vi "GenericDriveIO.vi"(0 "GenericDriveCommand":T1="DePowerMotor", 2 "Channel Name":string, 4 "String Value":string, 6 "Numeric Value":dbl format="%.2f", 8 "Address":u8, 9 "Type":string="ParkerX", 10 "Port Name":string) -> (5 "String Reply":string, 7 "Numeric Reply":sgl format="%.2f")   [LabVIEW 2014]
uses:
  GenericDriveCommand.ctl
  PARKER X/X-_commands.ctl
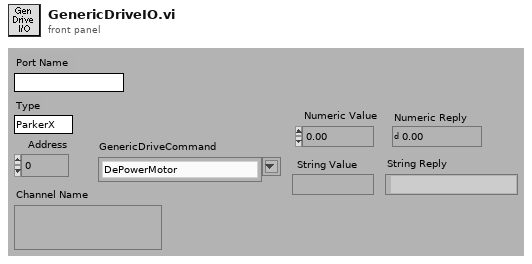
[diagram p1: front panel]
types:
  T1 = typedef "GenericDriveCommand.ctl" = string
  T2 = typedef "X-_commands.ctl" = enum16{"A-    Acceleration (rps)", "B-    Buffer Status", "C-    Continue", "CG-  Correction Gain", "CR-  Cariage Return", "D-    Distance (pulses)", "DB-  Dead Band (encoder steps)", "DW- Deadband Window (encoder steps)", "E-    Enable Communications", "ER-  Encoder Resolution (steps/rev)", "F-    Disable Communications", "FS-  Encoder Functions Report", "FSA- Incremental/Absolute (0/1)", "FSB- Motor/Encoder Step Mode (0/1)", "FSC- Enable/Disable Position Maint. (1/0)", "FSD- Stop/Continue on Stall (1/0)", "FSE- Activate o/p1 on Stall (1/0)", "FSF- Stop Motion on Trig3 (1/0)", "FSG- Activate o/p2 in Deadband (1/0)", "FSH- Enable Stall Detect (1/0)", "G- Go", "GH- Go Home and Zero (+/-V)", "^H- Delete ", "H- Direction Reverse/CCW/CW (0,1,2)", "IS- Input Status", "K- Kill", "L- Loop (n)", "LD- Limit DISABLE (0-none,1-CW,2-CCW,3-Both)", "LF- Line Feed", "MC- Mode Continuous", "MN- Mode Normal", "MPA- Motor Postion Absolute", "MPI- Motor Position Incremental", "MR- Motor Resolution (Drive Steps/rev)", "N- End of Loop", "O- Output (00,01,10,11)", "OS- Report Homing Setup", "OSA- NO/NC Limits (1/0)", "OSB- Back Up to Home/Edge? (0/1)", "OSC- NO/NC Home Switch (1/0)", "OSD- Enable Encoder Z for Home (0/1)", "OSH- Reference Edge for Home CW/CCW (0/1)", "PR- Report ABSOLUTE Position", "PS- Pause until Continue", "PX- Report Absolute ENCODER Position", "PZ- Zero Absolute Counter", "\"- Quote (17 ASCII +Space)", "Q- Enter/Exit Velocity Profiling (1/0)", "R- Request Indexer Status", "RA- Report Limit Switch Status", "RB- Report Loop, Pause, Shutdown, Trigger Status", "RC- Report Closed Loop Status", "RM- Velocity Streaming Rate Multiplier (000-FFF)", "RV- Report Revision Level", "S- Controlled Stop", "SN- Debounce (1-1000ms)", "SS- Report Software Switch Status", "SSA- Disable RS232 Echo (1/0)", "SSG- Clear/Save Command Buffer on Limit (0/1)", "SSH- Clear/Save Command Buffer on Stop (0/1)", "ST- Shutdown (1/0)", "SV- Servoing Setting (0,1,2,3)", "T- Time Delay (0.01-99999.99)", "TR- Wait for Trigger High/Low/Ignore (1/0/X)", "TS- Report Trigger Status", "U- Pause after Move Until Continue", "V- Velocity (0.01-50.00 revs/sec)", "W1- Report Relative Position <Signed Binary>", "W3- Report Relative Position <Hexadecimal>", "Y- Abort Loop at N", "Z-    Reset to Defaults", "#-    Disable/Set Soft Addresses (0/1-255)"}
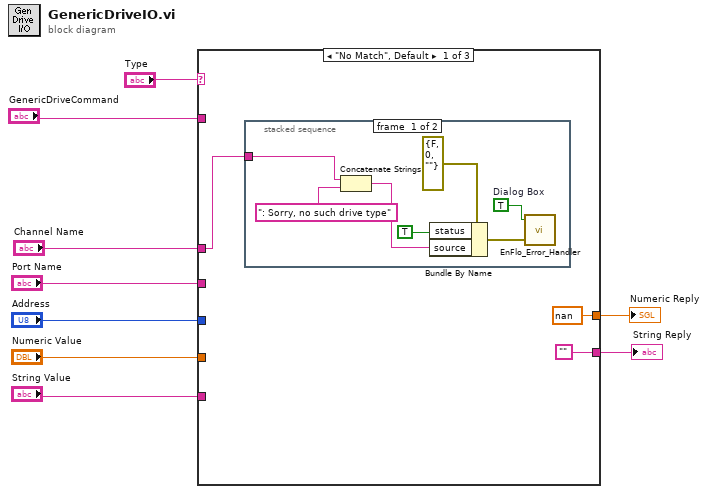
[diagram p0: block diagram]
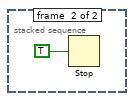
[diagram p2: hidden frame]
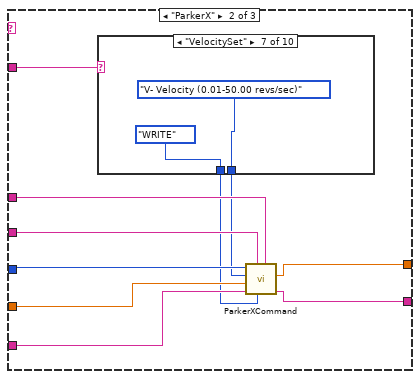
[diagram p3: hidden frame]
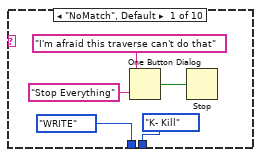
[diagram p4: hidden frame]
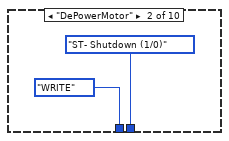
[diagram p5: hidden frame]
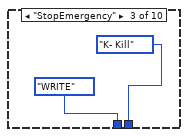
[diagram p6: hidden frame]
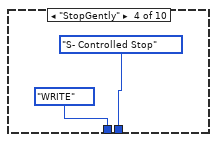
[diagram p7: hidden frame]
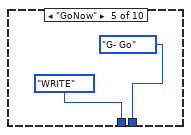
[diagram p8: hidden frame]
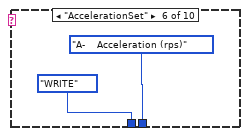
[diagram p9: hidden frame]
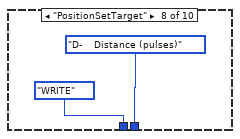
[diagram p10: hidden frame]
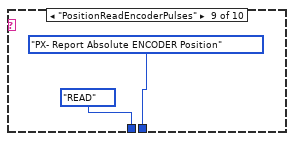
[diagram p11: hidden frame]
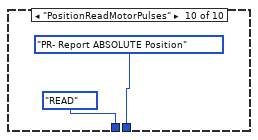
[diagram p12: hidden frame]
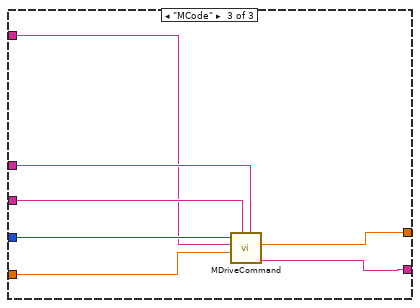
[diagram p13: hidden frame]
diagram:
  n1 = case shown="\"No Match\", Default" "Type" {
    tunnel: "Port Name" -> [_ w28 w58]
    tunnel: "Address" -> [_ w27 w60]
    tunnel: "Numeric Value" -> [_ w25 w56]
    tunnel: "String Value" -> [_ w24 _]
    tunnel: "Channel Name" -> [w10 w29 w59]
    tunnel: [nan ("Numeric Reply") w23 w55] -> w4
    tunnel: ["" w22 w54] -> w3
    tunnel: "GenericDriveCommand" -> [_ w30 w57]
    frame "No Match", Default {
      n2 = stacked-sequence {
        tunnel: w10 -> [w13 _]
        frame #0 {
          w14 = TRUE  # Dialog Box
          n3 = Concatenate Strings(w13, ": Sorry, no such drive type") -> (w15:string)
          n4 = Bundle By Name(cluster=errorcluster {"status"=FALSE, "code"=0, "source"=""} ("error in (no error)"), "status"=TRUE ("Bundle Element"), "source"=w15) -> (w18:errorcluster)
          n5 = call "EnFlo_Error_Handler.vi"("error in (no error)"=w18, "Dialog Box (T)"=w14) -> ()  [unwired: 1 in, 3 out]
        }
        frame #1 {
          n6 = Stop(stop? (T)=TRUE) -> ()
        }
      }
    }
    frame "ParkerX" {
      n7 = case shown="\"VelocitySet\"" w30 {
        tunnel: [X-_commands."K- Kill" ("COMMAND") X-_commands."ST- Shutdown (1/0)" ("COMMAND") X-_commands."K- Kill" ("COMMAND") X-_commands."S- Controlled Stop" ("COMMAND") X-_commands."G- Go" ("COMMAND") X-_commands."A-    Acceleration (rps)" ("COMMAND") X-_commands."V- Velocity (0.01-50.00 revs/sec)" ("COMMAND") X-_commands."D-    Distance (pulses)" ("COMMAND") X-_commands."PX- Report Absolute ENCODER Position" ("COMMAND") X-_commands."PR- Report ABSOLUTE Position" ("COMMAND")] -> w26
        tunnel: [enum16{"READ", "WRITE"}."WRITE" ("R/W") enum16{"READ", "WRITE"}."WRITE" ("R/W") enum16{"READ", "WRITE"}."WRITE" ("R/W") enum16{"READ", "WRITE"}."WRITE" ("R/W") enum16{"READ", "WRITE"}."WRITE" ("R/W") enum16{"READ", "WRITE"}."WRITE" ("R/W") enum16{"READ", "WRITE"}."WRITE" ("R/W") enum16{"READ", "WRITE"}."WRITE" ("R/W") enum16{"READ", "WRITE"}."READ" ("R/W") enum16{"READ", "WRITE"}."READ" ("R/W")] -> w21
        frame "NoMatch", Default {
          n8 = One Button Dialog(message="I'm afraid this traverse can't do that", button name ("OK")="Stop Everything") -> (true=w33:bool)
          n9 = Stop(stop? (T)=w33) -> ()
        }
        frame "DePowerMotor" {
        }
        frame "StopEmergency" {
        }
        frame "StopGently" {
        }
        frame "GoNow" {
        }
        frame "AccelerationSet" {
        }
        frame "VelocitySet" {
        }
        frame "PositionSetTarget" {
        }
        frame "PositionReadEncoderPulses" {
        }
        frame "PositionReadMotorPulses" {
        }
      }
      n10 = call "ParkerXCommand.vi"("Channel Name"=w29, "R/W"=w21, "Port Name"=w28, "String Value"=w24, "Numeric Value"=w25, "COMMAND"=w26, "Address"=w27) -> ("String Reply"=w22:string, "Numeric Reply"=w23:dbl)  [unwired: 2 out]
    }
    frame "MCode" {
      n11 = call "MDriveCommand.vi"("Channel Name"=w59, "Port Name"=w58, "Numeric Value"=w56, "MDriveCommand"=w57, "Address"=w60) -> ("String Reply"=w54:string, "Numeric Reply"=w55:dbl)  [unwired: 2 in, 2 out]
    }
  }
  "String Reply" <- w3
  "Numeric Reply" <- w4
